vi "Initialize.vi"(8 "error in (no error)":errorcluster, 11 "MASTER in":refnum<class "MASTER.lvclass">) -> (0 "error out":errorcluster, 3 "MASTER out":refnum<class "MASTER.lvclass">)   [LabVIEW 2014, in "Files Library.lvlib" / "Master.lvclass"]
uses:
  MASTER/MASTER.lvclass
  CONTROL/statedef.ctl
  MASTER/MASTER.lvclass/MASTER.ctl
  CONTROL/CONTROL LIBRARY.lvlib
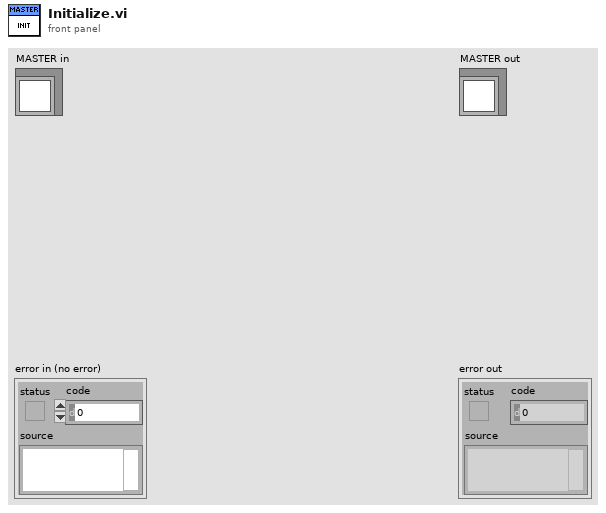
[diagram p1: front panel]
types:
  T1 = typedef "CONTROL LIBRARY.lvlib/statedef.ctl" = cluster{"State":string, "Data":variant}
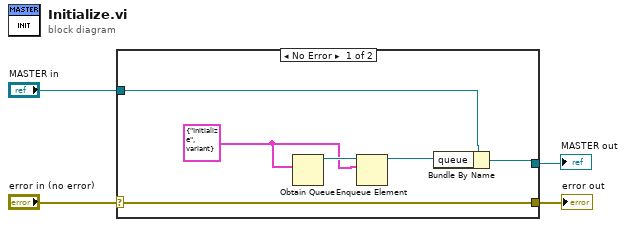
[diagram p0: block diagram]
diagram:
  n1 = case shown="No Error" "error in (no error)" {
    selector: "error in (no error)" -> [w10 w12]
    tunnel: [w10 w12] -> w3
    tunnel: [w5 w11] -> w1
    tunnel: "MASTER in" -> [w6 w11]
    frame No Error {
      w7 = T1 {"State"="Initialize", "Data"=variant} ("StateDatas")
      n2 = Obtain Queue(element data type=w7) -> (queue out=w9:refnum<queue>)  [unwired: 4 in, 2 out]
      n3 = Enqueue Element(queue=w9, element=w7) -> (queue out=w8:refnum<queue>)  [unwired: 2 in, 2 out]
      n4 = Bundle By Name(cluster=w6, "queue"=w8) -> (w5:refnum<class "MASTER.lvclass">)
    }
    frame Error {
    }
  }
  "error out" <- w3
  "MASTER out" <- w1
